vi "Example Callback - Color Callback.vi"(4 "Color":refnum<user-event>, 5 "Event Data":T1, 6 "Control Ref":refnum<k24>, 7 "Event Common Data":T2) -> ()   [LabVIEW 2010]
uses:
  C:/tf/play/labview/Tinkerforge.dll
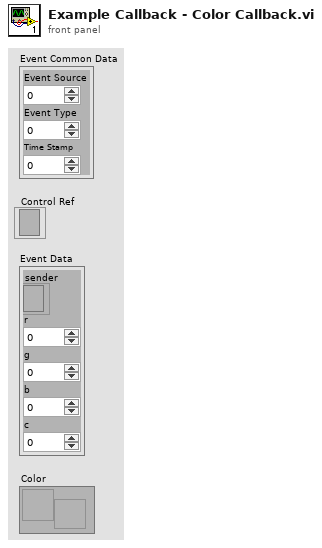
[diagram p1: front panel]
types:
  T1 = cluster{"sender":refnum<k24>, "r":i32, "g":i32, "b":i32, "c":i32}
  T2 = cluster{"Event Source":i32, "Event Type":u32, "Time Stamp":u32}
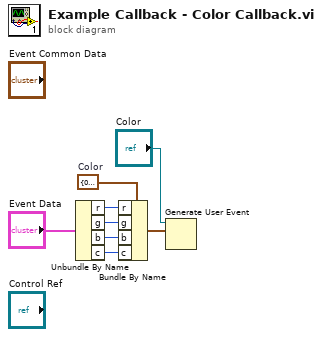
[diagram p0: block diagram]
diagram:
  w8 = cluster{"r":i32, "g":i32, "b":i32, "c":i32} {"r"=0, "g"=0, "b"=0, "c"=0}  # Color
  n1 = Unbundle By Name("Event Data") -> ("r"=w6:i32, "g"=w5:i32, "b"=w4:i32, "c"=w3:i32)
  n2 = Bundle By Name(cluster=w8, "r"=w6, "g"=w5, "b"=w4, "c"=w3) -> (w2:cluster{"r":i32, "g":i32, "b":i32, "c":i32})
  n3 = Generate User Event(user event="Color", event data cluster=w2) -> ()  [unwired: 1 in, 2 out]
